vi "AO Python Read TCP Data.vi"(0 "Connection ID":refnum<k5>, 11 "Error":errorcluster, 13 "Timeout (ms)":i32=5000) -> (4 "Connection ID (Dup)":refnum<k5>, 8 "Read String":string, 15 "Error Out":errorcluster)   [LabVIEW 2016]
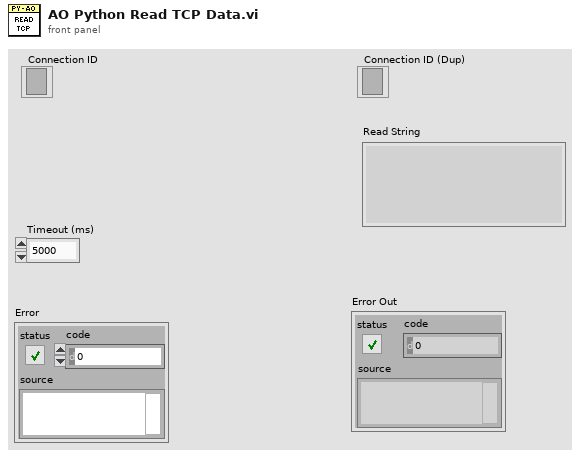
[diagram p1: front panel]
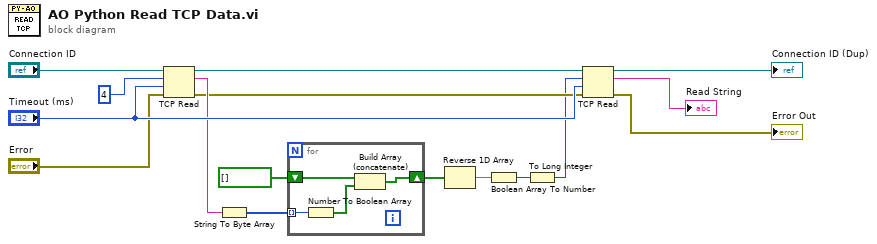
[diagram p0: block diagram]
diagram:
  n1 = TCP Read(connection ID="Connection ID", bytes to read=4, error in (no error)="Error", 9:"Timeout (ms)") -> (connection ID out=w6:refnum<k5>, data out=w11:string, error out=w5:errorcluster)  [unwired: 1 in]
  n2 = String To Byte Array(string=w11) -> (unsigned byte array=w10:u8[])
  n3 = for {
    tunnel: w10 -> [w20] mode=indexing
    shift-right: [w17] -> w8
    shift-left: bool[] [] -> [w19]
    n4 = Number To Boolean Array(number=w20) -> (Boolean array=w18:bool[])
    n5 = Build Array (concatenate)(w19, w18) -> (w17:bool[])
  }
  n6 = Reverse 1D Array(array=w8) -> (reversed array=w3:bool[])
  n7 = Boolean Array To Number(Boolean array=w3) -> (number=w7:u32)
  n8 = To Long Integer(number=w7) -> (32bit integer=w4:i32)
  n9 = TCP Read(connection ID=w6, bytes to read=w4, error in (no error)=w5, 9:"Timeout (ms)") -> (connection ID out=→"Connection ID (Dup)":refnum<k5>, data out=→"Read String":string, error out=→"Error Out":errorcluster)  [unwired: 1 in]
